vi "Write Headers.vi"(8 "error in (no error)":errorcluster, 9 "Header Values":string[](array[string]), 10 "Header Names":string[](array[string]), 11 "Linked List Header in":refnum<class "Linked List Header.lvclass">) -> (0 "error out":errorcluster, 3 "Linked List Header out":refnum<class "Linked List Header.lvclass">)   [LabVIEW 2020, in "Linked Lists.lvlib" / "Linked List Header.lvclass"]
uses:
  <vilib>/gpm_packages/@cs/linked-list/Source/Linked List/Linked List Header/Linked List Header.lvclass
  <vilib>/gpm_packages/@cs/linked-list/Source/Linked List/Linked List Header/Linked List Header.lvclass/Linked List Header.ctl
  <vilib>/gpm_packages/@cs/lookup-table/Source/LookupTable/LookupTable.lvclass/LookupTable.ctl
  a942fcd2-d4e0-4839-acba-2f659c0cf458.vi
  <vilib>/gpm_packages/@cs/lookup-table/Source/LookupTable/Read Table Reference.vi
  a942fcd2-d4e0-4839-acba-2f659c0cf458.vi/be145551-74e4-4a64-a602-a57447c4dae2.vi
  <vilib>/gpm_packages/@cs/lookup-table/Source/LookupTable/LookupTable.lvclass
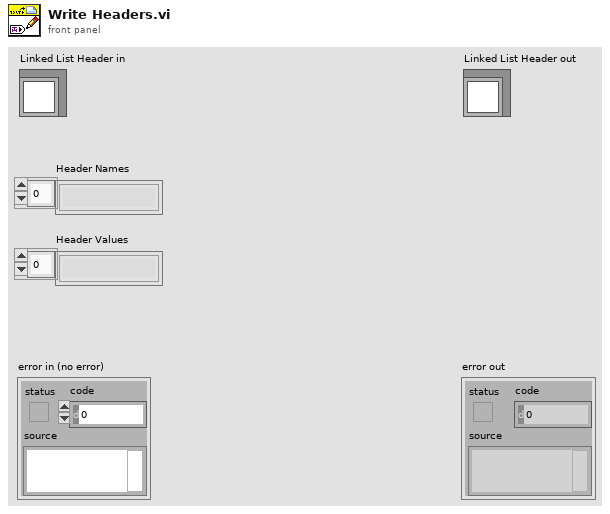
[diagram p1: front panel]
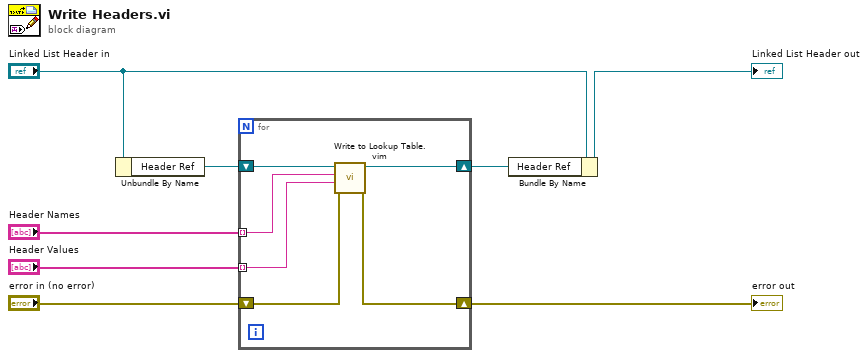
[diagram p0: block diagram]
diagram:
  n1 = Unbundle By Name("Linked List Header in") -> ("Header Ref"=w8:refnum<data-value>)
  n2 = for {
    shift-right: [w13] -> w7
    shift-left: w8 -> [w14]
    shift-right: [w11] -> w3
    shift-left: "error in (no error)" -> [w12]
    tunnel: "Header Names" -> [w10] mode=indexing
    tunnel: "Header Values" -> [w9] mode=indexing
    n3 = call "Write to Lookup Table.vim"("error in (no error)"=w12, "Item"=w9, "Item Name"=w10, "LookupTable Reference"=w14) -> ("error out"=w11:errorcluster, "LookupTable Reference Out"=w13:refnum<data-value>)  [unwired: 5 in, 1 out]
  }
  "error out" <- w3
  n4 = Bundle By Name(cluster="Linked List Header in", "Header Ref"=w7) -> (→"Linked List Header out":refnum<class "Linked List Header.lvclass">)
